vi "Read Author.vi"(8 "error in (no error)":errorcluster, 11 "Lv Proj Document Type:TAF Proj Config in":refnum<class "TAF Proj Config.lvclass">) -> (0 "error out":errorcluster, 2 "Author":string, 3 "Lv Proj Document Type:TAF Proj Config out":refnum<class "TAF Proj Config.lvclass">)   [LabVIEW 2021, in "TAF Proj Document Type.lvlib" / "TAF Proj Config.lvclass"]
uses:
  <vilib>/Wovalab/AntiDoc/Document Type/Add-ons/LabVIEW TAF Project/TAF Proj Config/TAF Proj Config.lvclass
  <vilib>/Wovalab/AntiDoc/Document Type/Add-ons/LabVIEW TAF Project/TAF Proj Config/TAF Proj Config.lvclass/TAF Proj Config.ctl
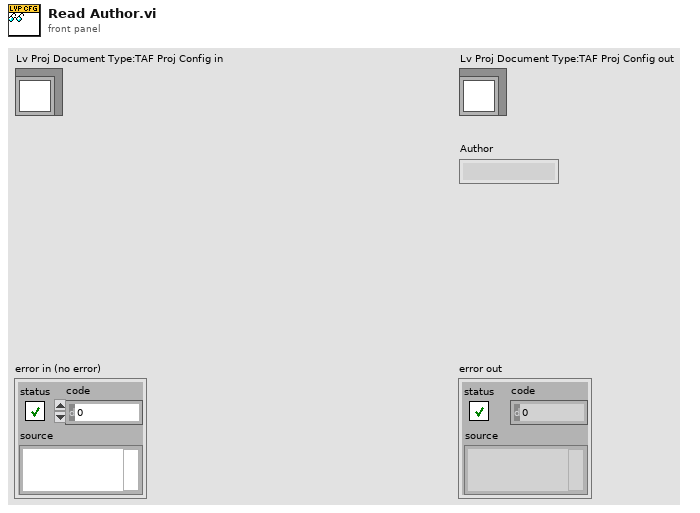
[diagram p1: front panel]
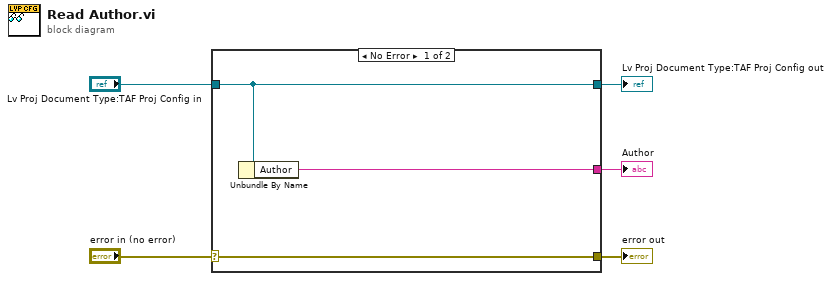
[diagram p0: block diagram]
diagram:
  n1 = case shown="No Error" "error in (no error)" {
    selector: "error in (no error)" -> [w8 w9]
    tunnel: [w8 w9] -> w4
    tunnel: [w7 w10] -> w2
    tunnel: "Lv Proj Document Type:TAF Proj Config in" -> [w7 w10]
    tunnel: [w6 _] -> w1
    frame No Error {
      n2 = Unbundle By Name(w7) -> ("Author"=w6:string)
    }
    frame Error {
    }
  }
  "error out" <- w4
  "Lv Proj Document Type:TAF Proj Config out" <- w2
  "Author" <- w1
